vi "Timestamp.vi"(0 "error in (no error)":errorcluster) -> (1 "current time (time stamp)":timestamp, 2 "current time (sec)":dbl, 3 "error out":errorcluster)   [LabVIEW 2019]
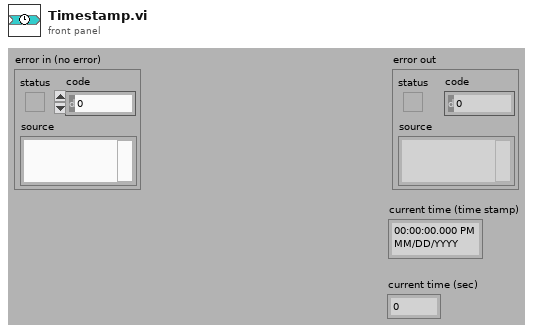
[diagram p1: front panel]
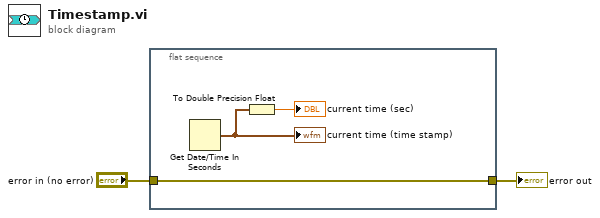
[diagram p0: block diagram]
diagram:
  n1 = flat-sequence {
    tunnel: "error in (no error)" -> [w5]
    tunnel: [w5] -> w1
    frame #0 {
      n2 = Get Date/Time In Seconds() -> (seconds since 1Jan1904=w4:timestamp)
      "current time (time stamp)" <- w4
      n3 = To Double Precision Float(number=w4) -> (double precision float=→"current time (sec)":dbl)
    }
  }
  "error out" <- w1
